vi "tsfifo_read_canfd_tx_buffer_frame_count.vi"(8 "error in (no error)":errorcluster caption="错误输入（无错误）", 10 "AIdxChn":i32, 11 "路径输入":path) -> (0 "error out":errorcluster caption="错误输出", 1 "ACount out":i32, 2 "function return":i32, 3 "路径输出":path)   [LabVIEW 2014]
doc: "Function Name :\nint tsfifo_read_canfd_buffer_frame_count(int AIdxChn, ref int ACount)\nFunction Introduction :\nRead the number of canfd transmission buffer messages\nCall location :\nAfter loading the database\ninput parameter :\nAChn: Channel\nACount: The number of frames returned\nReturn value :\n==0: Execution successful\nOther values: Query error code"
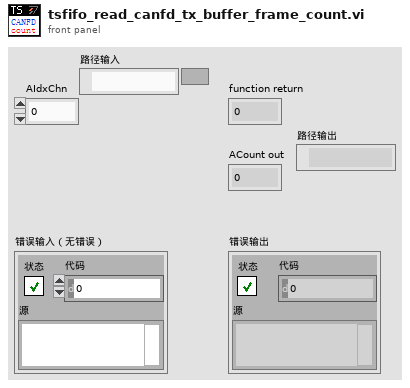
[diagram p1: front panel]
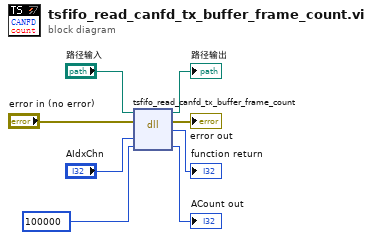
[diagram p0: block diagram]
diagram:
  n1 = dll-call lib="D:/Work/LabVIEW Code/TSMaster Labview SDK/LabVIEW/LabVIEW-TSMasterAPI_CLN/TSMasterAPI_LabVIEW-2024-09-06 14-39-20/Not_organized_vi/TSMaster.*" fn="tsfifo_read_canfd_tx_buffer_frame_count"(path in="路径输入", error in="error in (no error)", "AIdxChn"="AIdxChn", "ACount"=100000) -> (path out=→"路径输出":path, error out=→"error out":errorcluster, "返回类型"=→"function return":i32, "ACount"=→"ACount out":i32)  [unwired: 2 in]
